vi "Cub Meaasure PD FGV.vi"(0 "Action":T3=enum."Write", 1 "AddTable 6":string[][](table)=[["Tray Barcode", ""], ["PCBA BARCODE", ""], ["硬體(Tool初始化)", ""], ["company(Tool初始化)", ""], ["耗電流 uA(電流表)", ""], ["電池負載電壓", ""], ["晶片ID(Tool FORMAT)", ""], ["雷雕ID(TOOl scan、藍芽接收器)", ""], ["Format(Tool FORMAT)", ""], ["Programe(Tool Programe)", ""], ["MAC(藍芽接收器)", ""], ["ID(藍芽接收器)", ""], ["KPA(藍芽接收器)", ""], ["溫度(藍芽接收器)", ""], ["SENSOR電池電壓(藍芽接收器)", ""], ["RSSI(藍芽接收器)", ""], ["SensorType_315(FSK scan)", ""], ["FSKsnVol_315(FSK scan)", ""], ["FSKscanl_315(FSK scan)", ""], ["P_315(Tool FSK scan)", ""], ["T_315(Tool FSK scan)", ""], ["SensorType_433(ASK scan)", ""], ["ASKsnVol_433(ASK scan)", ""], ["ASKscan_433(ASK scan)", ""], ["P_433(ASK scan)", ""], ["T_433(ASK scan)", ""], ["測高Data", ""]], 2 "Save low Index":T2, 3 "Save Col Index":T1, 4 "DataIn":string, 5 "SN":string, 6 "Table Load":cluster{"Table Control":string[][]}[](array[cluster]), 7 "error in (no error)":errorcluster) -> (12 "條碼的Index":i32, 13 "Read SN Table":string[][](array[string]), 14 "Total Table":cluster{"Table Control":string[][]}[](array[cluster]), 15 "Barcode Array":string[](array[string]), 16 "Read Index Data":string, 17 "Read first table":string[][](array[string]), 18 "Barcode重複":bool, 19 "error out":errorcluster)   [LabVIEW 2019]
uses:
  Ctrl/MeasureDisplayTab.ctl
  Ctrl/Table Save.ctl
  Ctrl/PD Table Save Low Index.ctl
  Ctrl/PD Table Save Col Index.ctl
  9377167a-9215-4fe1-b1d7-405c4c1bac97.vi
  09652be0-0e8a-482c-be89-5823cf7997f4.vi
  <vilib>/Utility/xml.llb/Write to XML File(string).vi
  <vilib>/Utility/xml.llb/Read From XML File(string).vi
panel:
  in  "all rows 2":string[][](array[string])=[["", "", "CE18052500414910267_C2DC49A2(一般模式及藍芽模式 MES的LOG格式_半成品格式說明)", "", "", "", "", "", "", "", "", "", "", "", "", "", "", "", "", "", "", "", "", "", "", "", "", "", "", "", "", "", "", "", "", "", "", "", "", "", "", "", "", "", "", ""], ["", "", "PCBA SN", "scan 半成品 ID_1(scan )", "半成品 Waste_Time", "半成品 Result", "半成品 DateTime", "433半成品 版本", "433半成品 company", "433半成品 FF", "433半成品 SensorType", "433半成品 BattVol", "433半成品 ASKsnVOL", "433半成品 ID_2", "433半成品 Format", "433半成品 Programe", "433半成品 ASKscan", "433半成品 FSKscan", "433半成品 Batt", "433半成品 SN", "433半成品 Ptest", "433半成品 Ttest", "433半成品 P ", "433半成品 T", "433半成品 結果", "433半成品 箱號", "不良代碼", "電流", "電池電壓", "315半成品 版本", "315半成品 company", "315半成品 FF", "315半成品 SensorType", "315半成品 BattVol", "315半成品 ASKsnVOL", "315半成品 ID_2", "315半成品 Format", "315半成品 Programe", "315半成品 ASKscan", "315半成品 FSKscan", "315半成品 Batt", "315半成品 SN", "315半成品 Ptest", "315半成品 Ttest", "315半成品 P ", "315半成品 T"], ["", "", "", "", "", "", "", "", "", "", "", "", "", "", "", "", "", "", "", "", "", "", "", "", "", "", "", "", "", "", "", "", "", "", "", "", "", "", "", "", "", "", "", "", "", ""], ["", "", "", "", "", "", "", "", "", "", "", "", "", "", "", "", "", "", "", "", "", "", "", "", "", "", "", "", "", "", "", "", "", "", "", "", "", "", "", "", "", "", "", "", "", ""], ["一般模式", "FORMAT", "", "x", "", "", "", "v", "v", "x", "v", "x", "x", "v", "v", "x", "x", "x", "v", "x", "x", "x", "x", "x", "", "x", "", "2站", "x", "v", "v", "x", "v", "x", "x", "v", "v", "x", "x", "x", "v", "x", "x", "x", "x", "x"], ["", "PROGRAM", "", "x", "", "", "", "v", "v", "x", "v", "x", "x", "v", "x", "v", "x", "x", "x", "x", "x", "x", "x", "x", "", "x", "", "x", "x", "v", "v", "x", "v", "x", "x", "v", "x", "v", "x", "x", "x", "x", "x", "x", "x", "x"], ["", "SCAN", "", "SCAN雷雕ID", "", "", "", "v", "v", "v", "v", "x", "ASK SCAN", "ASK SCAN", "x", "x", "ASKscan", "x", "x", "ASKscan", "ASKscan", "ASKscan", "ASKscan", "ASKscan", "", "x", "", "x", "電子負載電壓", "v", "v", "v", "v", "x", "FSKSCAN", "FSKSCAN", "x", "x", " ASKscan", "FSKscan", "x", "FSKscan", "FSKscan", "FSKscan", "FSKscan", "FSKscan"], ["", "", "", "", "", "", "", "", "", "", "", "", "", "", "", "", "", "", "", "", "", "", "", "", "", "", "", "", "", "", "", "", "", "", "", "", "", "", "", "", "", "", "", "", "", ""], ["藍芽模式", "FORMAT", "", "x", "", "", "", "x", "v", "x", "v", "x", "x", "v", "v", "x", "x", "x", "x", "x", "x", "x", "x", "x", "", "x", "", "2站", "x", "x", "x", "x", "x", "x", "x", "x", "x", "x", "x", "x", "x", "x", "x", "x", "x", "x"], ["", "PROGRAM", "", "x", "", "", "", "x", "v", "x", "v", "x", "x", "v", "x", "v", "x", "x", "x", "x", "x", "x", "x", "x", "", "x", "", "x", "x", "x", "x", "x", "x", "x", "x", "x", "x", "x", "x", "x", "x", "x", "x", "x", "x", "x"], ["", "SCAN", "", "藍芽接收器 ID", "", "", "", "藍芽接收器 MAC", "v", "v", "v", "藍芽接收器電池電壓", "藍芽接收器RSSI", "v", "x", "x", "x", "x", "x", "x", "x", "x", "藍芽接收器 KPA", "藍芽接收器 C", "", "x", "", "x", "電子負載電壓", "x", "x", "x", "x", "x", "x", "x", "x", "x", "x", "x", "x", "x", "x", "x", "x", "x"]]
  in  "AddTable 2":string[][](table)=[["PCBA BARCODE", ""], ["硬體(Tool初始化)", ""], ["company(Tool初始化)", ""], ["耗電流 uA(電流表)", ""], ["電池負載電壓", ""], ["晶片ID(Tool FORMAT)", ""], ["雷雕ID(TOOl scan、藍芽接收器)", ""], ["Format(Tool FORMAT)", ""], ["Programe(Tool Programe)", ""], ["MAC(藍芽接收器)", ""], ["ID(藍芽接收器)", ""], ["KPA(藍芽接收器)", ""], ["溫度(藍芽接收器)", ""], ["SENSOR電池電壓(藍芽接收器)", ""], ["RSSI(藍芽接收器)", ""], ["SensorType_315(FSK scan)", ""], ["FSKsnVol_315(FSK scan)", ""], ["FSKscanl_315(FSK scan)", ""], ["P_315(Tool FSK scan)", ""], ["T_315(Tool FSK scan)", ""], ["SensorType_433(ASK scan)", ""], ["ASKsnVol_433(ASK scan)", ""], ["ASKscan_433(ASK scan)", ""], ["P_433(ASK scan)", ""], ["T_433(ASK scan)", ""], ["測高Data", ""]]
  in  "Save low Index__":T4=enum."Format(Tool FORMAT)"
  in  "WriteTable":string[][](table)=[["PCBA BARCODE", ""], ["硬體(Tool初始化)", ""], ["company(Tool初始化)", ""], ["耗電流 uA(電流表)", ""], ["電池負載電壓", ""], ["晶片ID(Tool FORMAT)", ""], ["雷雕ID(TOOl scan、藍芽接收器)", ""], ["Format(Tool FORMAT)", ""], ["Programe(Tool Programe)", ""]]
  out "index of element":i32
  out "LOG":string[][](array[string])
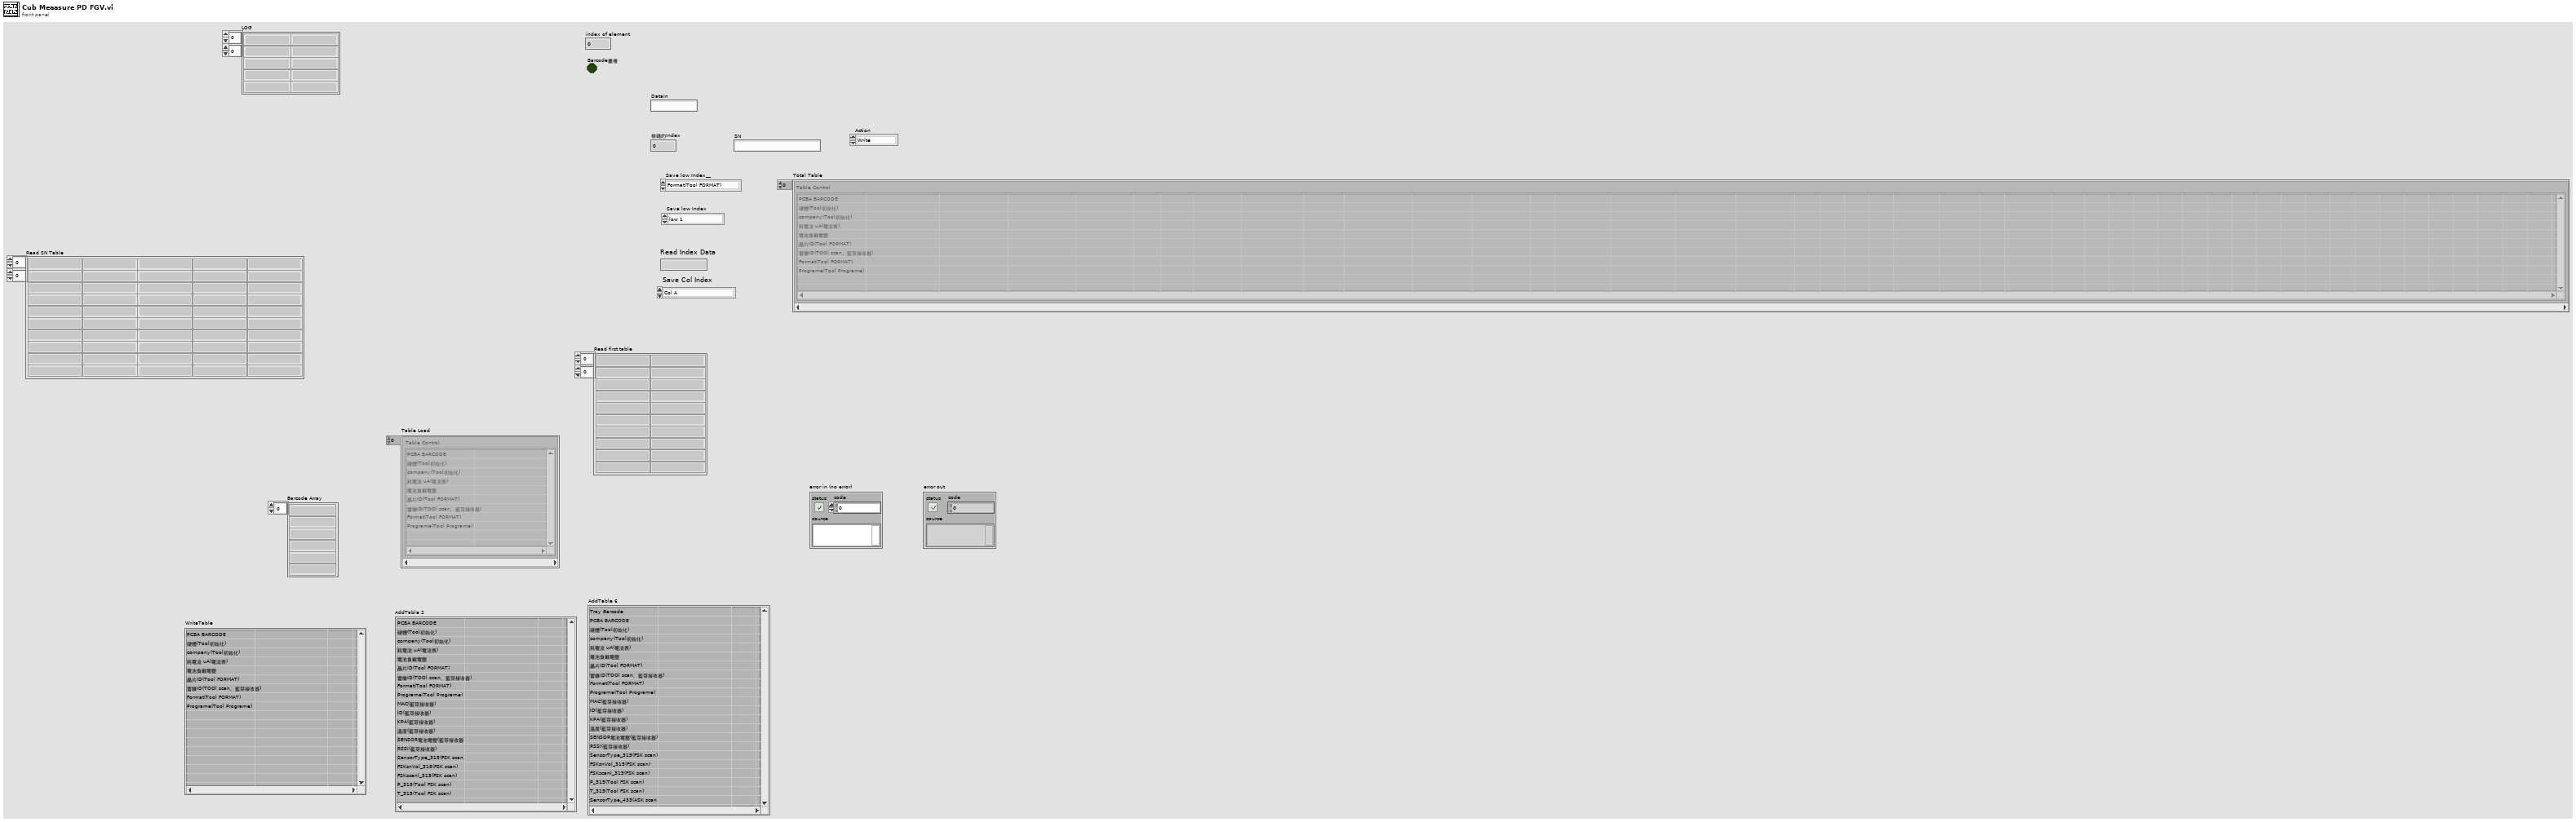
[diagram p1: front panel]
types:
  T1 = typedef "PD Table Save Col Index.ctl" = enum16{"Col A", "Col B", "PCBA SN_C", "scan 半成品 ID_1_D", "半成品 Waste_Time_E", "半成品 Result_F", "半成品 DateTime_G", "433半成品 版本_H", "433半成品 company_I", "433半成品 FF_J", "433半成品 SensorType_K", "433半成品 BattVol_L", "433半成品 ASKsnVOL_M", "433半成品 ID_2_N", "433半成品 Format_O", "433半成品 Programe_P", "433半成品 ASKscan_Q", "433半成品 FSKscan_R", "433半成品 Batt_S", "433半成品 SN_T", "433半成品 Ptest_U", "433半成品 Ttest_V", "433半成品 P_W", "433半成品 T_X", "433半成品 結果_Y", "433半成品 箱號_Z", "不良代碼_AA", "電流_AB", "電池電壓_AC", "315半成品 版本_AD", "315半成品 company_AE", "315半成品 FF_AF", "315半成品 SensorType_AG", "315半成品 BattVol_AH", "315半成品 ASKsnVOL_AI", "315半成品 ID_2_AJ", "315半成品 Format_AK", "315半成品 Programe_AL", "315半成品 ASKscan_AM", "315半成品 FSKscan_AN", "315半成品 Batt_AO", "315半成品 SN_AP", "315半成品 Ptest_AQ", "315半成品 Ttest_AR", "315半成品 P_AS", "315半成品 T_AT"}
  T2 = typedef "PD Table Save Low Index.ctl" = enum16{"low 1", "low 2", "low 3", "low 4", "一般模式F", "一般模式P", "一般模式S", "low 8", "藍芽模式F", "藍芽模式P", "藍芽模式S"}
  T3 = typedef "Table Save.ctl" = enum16{"initial", "Add", "Write", "Replace", "Delete", "REad", "RedTable", "Load"}
  T4 = typedef "MeasureDisplayTab.ctl" = enum16{"Tray Barcode", "PCBA BARCODE", "硬體(Tool初始化)", "company(Tool初始化)", "耗電流 uA(電流表)", "電池負載電壓", "晶片ID(Tool FORMAT)", "雷雕ID(TOOl scan、藍芽接收器)", "Format(Tool FORMAT)", "Programe(Tool Programe)", "MAC(藍芽接收器)", "ID(藍芽接收器)", "KPA(藍芽接收器)", "溫度(藍芽接收器)", "SENSOR電池電壓(藍芽接收器)", "RSSI(藍芽接收器)", "SensorType_315(FSK scan)", "FSKsnVol_315(FSK scan)", "FSKscanl_315(FSK scan)", "P_315(FSK scan)", "T_315(FSK scan)", "SensorType_433(ASK scan)", "ASKsnVol_433(ASK scan)", "ASKscan_433(ASK scan)", "P_433(ASK scan)", "T_433(ASK scan)", "測高Data"}
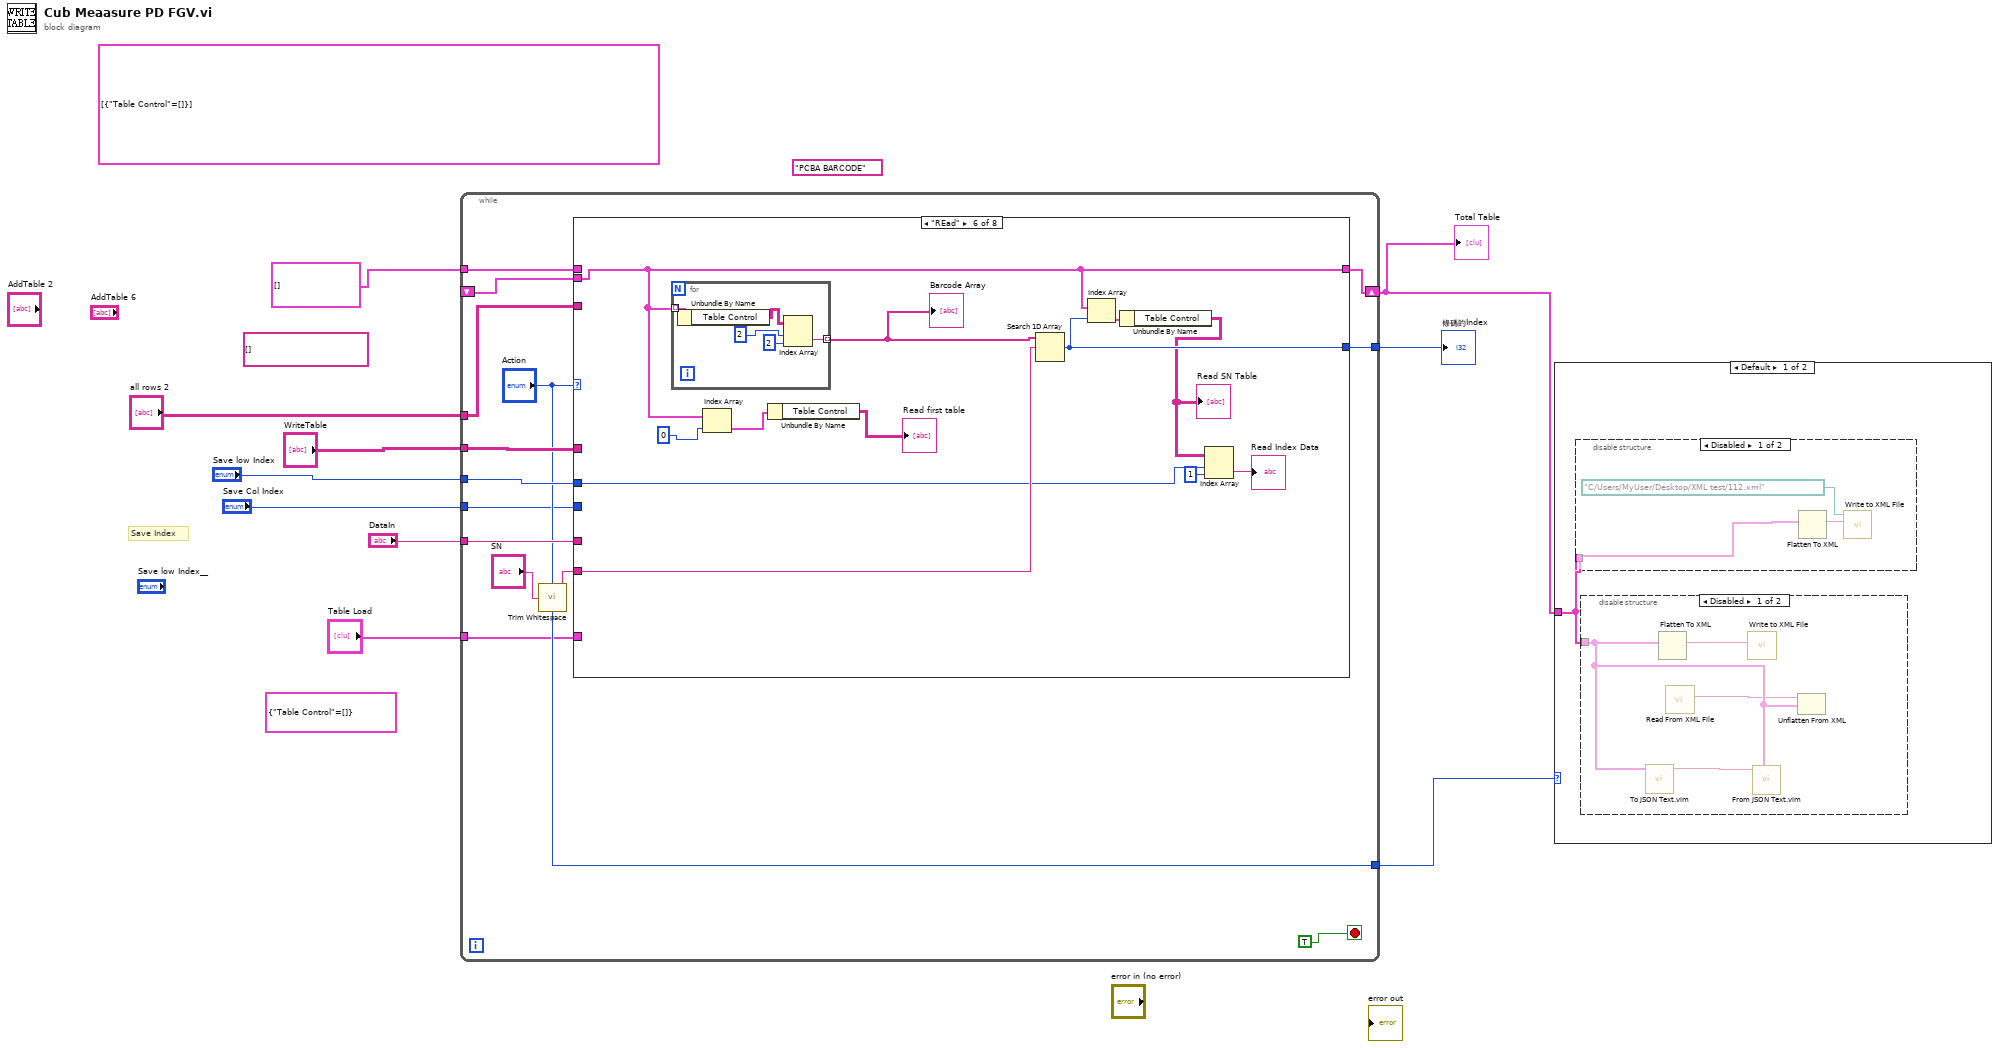
[diagram p0: block diagram]
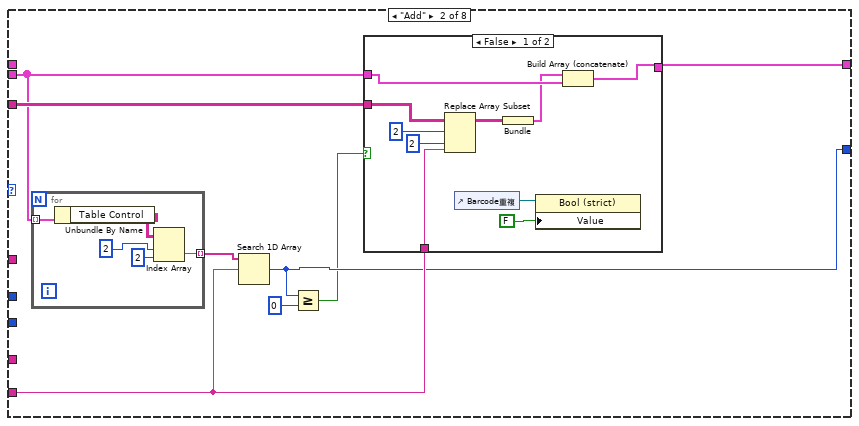
[diagram p6: hidden frame]
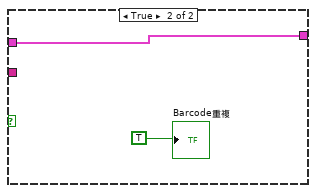
[diagram p7: hidden frame]
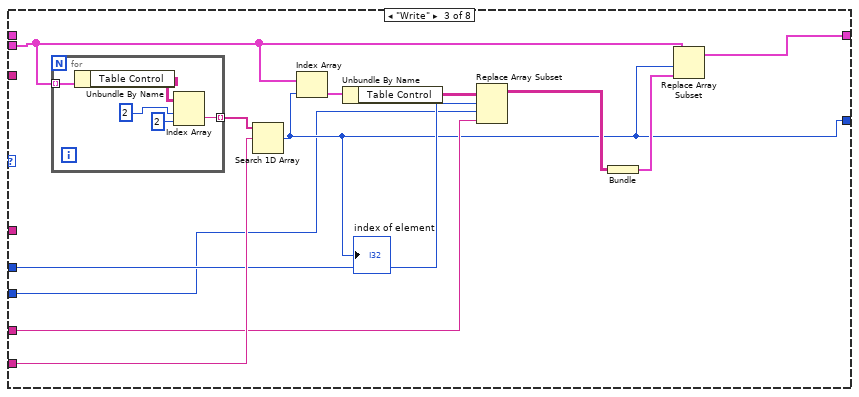
[diagram p8: hidden frame]
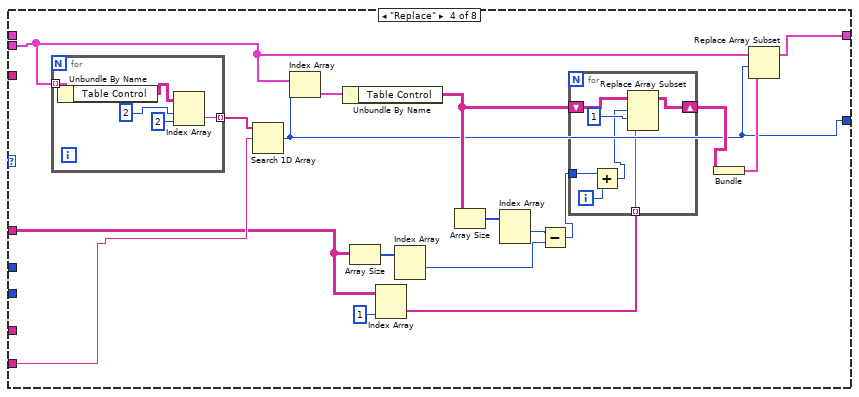
[diagram p9: hidden frame]
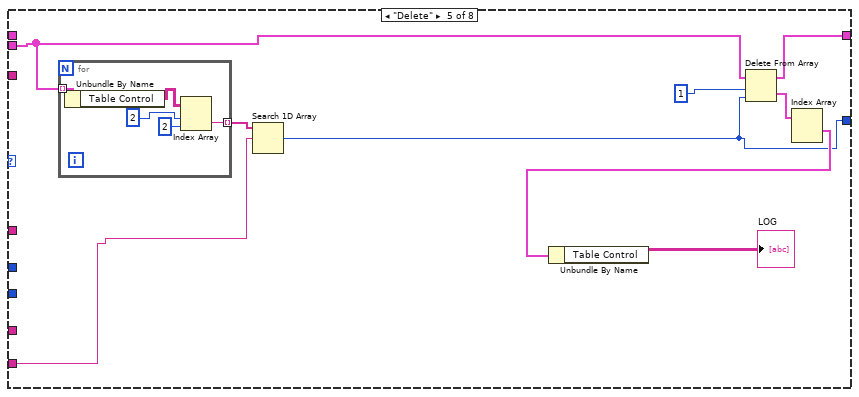
[diagram p10: hidden frame]
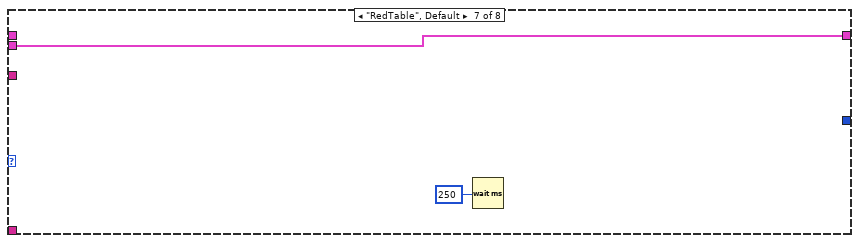
[diagram p11: hidden frame]
diagram:
  (unwired) cluster{"Table Control":string[][]} {"Table Control"=[]} ("Cluster")
  (unwired) "PCBA BARCODE"
  (unwired) string[][] [] ("Table Control")
  (unwired) cluster{"Table Control":string[][]}[] [{"Table Control"=[]}] ("Array 2")
  # "Save Index"
  n1 = while {
    tunnel: cluster{"Table Control":string[][]}[] [] ("Total Table") -> [w24]
    shift-right: [w23] -> w5
    shift-left: _ -> [w22]
    tunnel: "all rows 2" -> [w14]
    tunnel: "WriteTable" -> [w19]
    tunnel: ["Action"] -> w9
    tunnel: "Save low Index" -> [w21]
    tunnel: "DataIn" -> [w20]
    tunnel: [w17] -> w7
    tunnel: "Table Load" -> [w15]
    tunnel: "Save Col Index" -> [w13]
    stop <- TRUE stop-if-true
    n2 = call <vilib>:"Trim Whitespace.vi"("string"="SN") -> ("trimmed string"=w12:string)  [unwired: 1 in]
    n3 = case shown="\"REad\"" "Action" {
      tunnel: w24 -> [w25 _ _ _ _ _ _ _]
      tunnel: [w25 w33 w61 w82 w98 w120 w129 w130] -> w23
      tunnel: w14 -> [_ w31 _ _ _ _ _ _]
      tunnel: w22 -> [_ w29 w57 w80 w100 w120 w129 _]
      tunnel: w12 -> [_ w30 w59 w79 w104 w121 _ _]
      tunnel: w21 -> [_ _ w54 _ _ w113 _ _]
      tunnel: w20 -> [_ _ w53 _ _ _ _ _]
      tunnel: w19 -> [_ _ _ w69 _ _ _ _]
      tunnel: [_ w28 w52 w68 w97 w118 _ _] -> w17
      tunnel: w15 -> [_ _ _ _ _ _ _ w130]
      tunnel: w13 -> [_ _ w51 _ _ _ _ _]
      frame "initial" {
      }
      frame "Add" {
        n4 = for {
          tunnel: w29 -> [w50] mode=indexing
          tunnel: [w46] -> w32 mode=indexing
          n5 = Unbundle By Name(w50) -> ("Table Control"=w49:string[][])
          n6 = Index Array(array=w49, index (row)=2 ("disabled index (col)"), index (col)=2 ("disabled index (col)")) -> (element=w46:string)
        }
        n7 = Search 1D Array(1D array=w32, element=w30) -> (index of element=w28:i32)  [unwired: 1 in]
        n8 = Greater Or Equal?(x=w28, y=0) -> (x >= y?=w26:bool)
        n9 = case shown="False" w26 {
          tunnel: [w43 w45] -> w33
          tunnel: w31 -> [w40 _]
          tunnel: w30 -> [w39 _]
          tunnel: w29 -> [w35 w45]
          frame False {
            n10 = Replace Array Subset(array=w40, new element=w39, index (row)=2, index (col)=2) -> (w36:string[][])
            n11 = control-ref of="Barcode重複"() -> (w38:refnum<vi>)
            n12 = Bundle("all rows 2"=w36) -> (w34:cluster{"all rows 2":string[][]})  [unwired: 1 in]
            n13 = property class="Bool (strict)"(reference=w38, "Value"=FALSE) -> ()  [unwired: 1 in, 2 out]
            n14 = Build Array (concatenate)(w34, w35) -> (w43:cluster{"Table Control":string[][]}[])
          }
          frame True {
            "Barcode重複" <- TRUE
          }
        }
      }
      frame "Write" {
        n15 = for {
          tunnel: w57 -> [w67] mode=indexing
          tunnel: [w63] -> w62 mode=indexing
          n16 = Unbundle By Name(w67) -> ("Table Control"=w66:string[][])
          n17 = Index Array(array=w66, index (row)=2 ("disabled index (col)"), index (col)=2 ("disabled index (col)")) -> (element=w63:string)
        }
        n18 = Search 1D Array(1D array=w62, element=w59) -> (index of element=w52:i32)  [unwired: 1 in]
        "index of element" <- w52
        n19 = Index Array(array=w57, index=w52) -> (element=w58:cluster{"Table Control":string[][]})
        n20 = Unbundle By Name(w58) -> ("Table Control"=w56:string[][])
        n21 = Replace Array Subset(array=w56, new element=w53, index (row)=w54, index (col)=w51) -> (w55:string[][])
        n22 = Bundle("Table Control"=w55) -> (w60:cluster{"Table Control":string[][]})  [unwired: 1 in]
        n23 = Replace Array Subset(array=w57, new element=w60, index=w52) -> (w61:cluster{"Table Control":string[][]}[])
      }
      frame "Replace" {
        n24 = for {
          tunnel: w80 -> [w96] mode=indexing
          tunnel: [w92] -> w84 mode=indexing
          n25 = Unbundle By Name(w96) -> ("Table Control"=w95:string[][])
          n26 = Index Array(array=w95, index (row)=2 ("disabled index (col)"), index (col)=2 ("disabled index (col)")) -> (element=w92:string)
        }
        n27 = Search 1D Array(1D array=w84, element=w79) -> (index of element=w68:i32)  [unwired: 1 in]
        n28 = Index Array(array=w80, index=w68) -> (element=w83:cluster{"Table Control":string[][]})
        n29 = Unbundle By Name(w83) -> ("Table Control"=w72:string[][])
        n30 = Array Size(array=w69) -> (size(s)=w76:i32[])
        n31 = Index Array(array=w69, index (col)=1 ("disabled index (col)")) -> (element=w73:string[])  [unwired: 1 in]
        n32 = Index Array(array=w76) -> (element #1=w75:i32)  [unwired: 2 in, 1 out]
        n33 = Array Size(array=w72) -> (size(s)=w77:i32[])
        n34 = Index Array(array=w77) -> (element #1=w71:i32)  [unwired: 2 in, 1 out]
        n35 = Subtract(x=w71, y=w75) -> (x-y=w70:i32)
        n36 = for {
          shift-right: [w91] -> w78
          shift-left: w72 -> [w90]
          tunnel: w70 -> [w87]
          tunnel: w73 -> [w86] mode=indexing
          i -> [w88]
          n37 = Add(x=w87, y=w88) -> (x+y=w85:i32)
          n38 = Replace Array Subset(array=w90, new element=w86, index (row)=w85, index (col)=1 ("disabled index (col)")) -> (w91:string[][])
        }
        n39 = Bundle("Table Control"=w78) -> (w81:cluster{"Table Control":string[][]})  [unwired: 1 in]
        n40 = Replace Array Subset(array=w80, new element=w81, index=w68) -> (w82:cluster{"Table Control":string[][]}[])
      }
      frame "Delete" {
        n41 = for {
          tunnel: w100 -> [w110] mode=indexing
          tunnel: [w106] -> w105 mode=indexing
          n42 = Unbundle By Name(w110) -> ("Table Control"=w109:string[][])
          n43 = Index Array(array=w109, index (row)=2 ("disabled index (col)"), index (col)=2 ("disabled index (col)")) -> (element=w106:string)
        }
        n44 = Search 1D Array(1D array=w105, element=w104) -> (index of element=w97:i32)  [unwired: 1 in]
        n45 = Delete From Array(array=w100, length=1 ("index"), index=w97) -> (deleted portion=w103:cluster{"Table Control":string[][]}[], array with subset deleted=w98:cluster{"Table Control":string[][]}[])
        n46 = Index Array(array=w103) -> (element #1=w102:cluster{"Table Control":string[][]})  [unwired: 2 in, 1 out]
        n47 = Unbundle By Name(w102) -> ("Table Control"=→"LOG":string[][])
      }
      frame "REad" {
        n48 = for {
          tunnel: w120 -> [w127] mode=indexing
          tunnel: [w123] -> w122 mode=indexing
          n49 = Unbundle By Name(w127) -> ("Table Control"=w126:string[][])
          n50 = Index Array(array=w126, index (row)=2 ("disabled index (col)"), index (col)=2 ("disabled index (col)")) -> (element=w123:string)
        }
        "Barcode Array" <- w122
        n51 = Index Array(array=w120, index=0) -> (element=w117:cluster{"Table Control":string[][]})
        n52 = Unbundle By Name(w117) -> ("Table Control"=→"Read first table":string[][])
        n53 = Search 1D Array(1D array=w122, element=w121) -> (index of element=w118:i32)  [unwired: 1 in]
        n54 = Index Array(array=w120, index=w118) -> (element=w119:cluster{"Table Control":string[][]})
        n55 = Unbundle By Name(w119) -> ("Table Control"=w114:string[][])
        "Read SN Table" <- w114
        n56 = Index Array(array=w114, index (row)=w113, index (col)=1 ("disabled index (col)")) -> (element=→"Read Index Data":string)
      }
      frame "RedTable", Default {
        n57 = Wait (ms)(milliseconds to wait=250) -> ()  [unwired: 1 out]
      }
      frame "Load" {
      }
    }
  }
  "條碼的Index" <- w7
  "Total Table" <- w5
  n58 = case shown="Default" w9 {
    tunnel: w5 -> [w131 _]
    frame Default {
      n59 = disable-structure shown="Disabled" {
        disable-tunnel: w131 -> [w132 _]
        frame Disabled {
          n60 = Flatten To XML(anything=w132) -> (xml string=w134:string)
          n61 = call-poly <vilib>:"Write to XML File.vi"("XML Input"=w134, "XML File Path"=path "C:/Users/MyUser/Desktop/XML test/112.xml") -> ()  [unwired: 7 in, 3 out]
        }
        frame Enabled {
        }
      }
      n62 = disable-structure shown="Disabled" {
        disable-tunnel: w131 -> [w137 _]
        frame Disabled {
          n63 = call "To JSON Text.vim"("Anything"=w137) -> ("<JSON>"=w138:string)  [unwired: 9 in, 1 out]
          n64 = Flatten To XML(anything=w137) -> (xml string=w135:string)
          n65 = call-poly <vilib>:"Read From XML File.vi"() -> ("XML Elements"=w136:string)  [unwired: 9 in, 2 out]
          n66 = call-poly <vilib>:"Write to XML File.vi"("XML Input"=w135) -> ()  [unwired: 8 in, 3 out]
          n67 = call "From JSON Text.vim"("Data Type and Default Value"=w137, "JSON"=w138) -> ()  [unwired: 8 in, 2 out]
          n68 = Unflatten From XML(xml string=w136, type=w137) -> ()  [unwired: 1 in, 2 out]
        }
        frame Enabled {
        }
      }
    }
    frame "initial", "REad" {
    }
  }
